vi "jsq_save.vi"(5 "Save?":bool=TRUE, 8 "error in (no error)":errorcluster, 10 "SEQs":T1[](array[typedef]), 11 "Path":path=path "C:/Users/Adam/Desktop/test.json") -> (0 "error out":errorcluster, 1 "JSON string":string, 3 "json File Path(duplicate)":path)   [LabVIEW 2015, in "oskar_tools.lvlib"]
uses:
  oskar_tools.lvlib
  seq_line.ctl
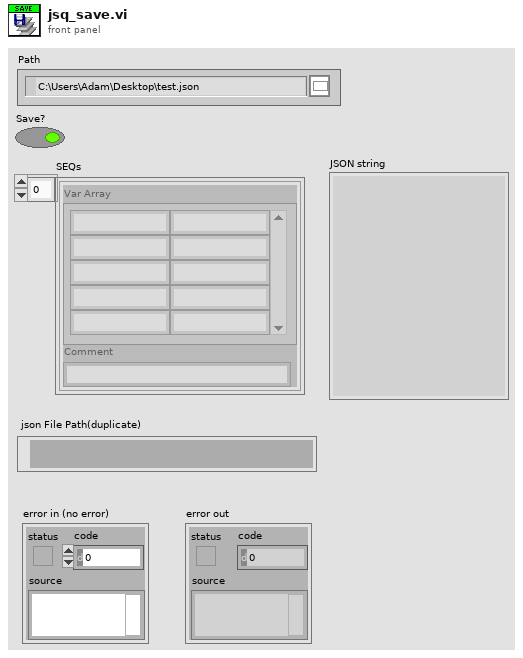
[diagram p1: front panel]
types:
  T1 = typedef "oskar_tools.lvlib/seq_line.ctl" = cluster{"Var Array":string[][], "Comment":string}
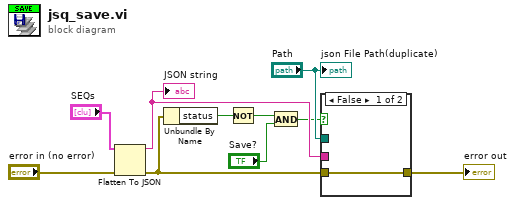
[diagram p0: block diagram]
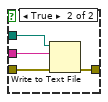
[diagram p2: hidden frame]
diagram:
  n1 = Flatten To JSON(anything="SEQs", error in (no error)="error in (no error)") -> (JSON string=w9:string, 11:w5:errorcluster)  [unwired: 1 in]
  "JSON string" <- w9
  n2 = Unbundle By Name(w5) -> ("status"=w2:bool)
  n3 = Not(x=w2) -> (.not. x?=w1:bool)
  n4 = And(x=w1, y="Save?") -> (x .and. y?=w3:bool)
  n5 = case shown="False" w3 {
    tunnel: w9 -> [_ w15]
    tunnel: [w11 w14] -> w8
    tunnel: "Path" -> [_ w13]
    tunnel: w5 -> [w11 w12]
    frame False {
    }
    frame True {
      n6 = Write to Text File(file (use dialog)=w13, text=w15, error in=w12) -> (error out=w14:errorcluster)  [unwired: 1 in, 2 out]
    }
  }
  "error out" <- w8
  "json File Path(duplicate)" <- "Path"
